vi "log.write.vi"(4 "Channel":string, 6 "Arguments":map{string, string}(c390), 7 "Time Stamp (now: system time)":timestamp format="%<%x %.3X>T", 8 "error in":errorcluster, 9 "Message":string, 10 "dataSourceRid":string, 11 "Nominal Client in":refnum<class "Nominal Client.lvclass">) -> (0 "error out":errorcluster, 3 "Nominal Client out":refnum<class "Nominal Client.lvclass">)   [LabVIEW 2020, in "Nominal Client.lvclass"]
doc: "Synchronously writes logs to a Nominal data source.\n\nMessage (required, string) The log content describing the event. Can include placeholder tokens for dynamic values.\n\nArguments (optional)\nKey-value pairs providing structured context data or filling message placeholders.\n\nChannel (optional, string, defaults to \"logs\") Logical grouping to organize logs by source, type, or system component for filtering and analysis."
uses:
  Nominal Client.lvclass
  <vilib>/Utility/error.llb/Error Cluster From Error Code.vi
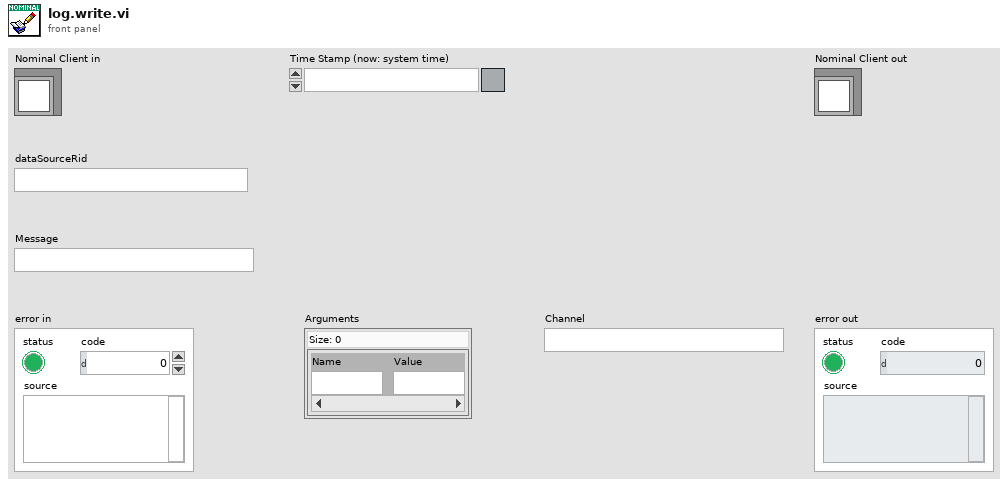
[diagram p1: front panel]
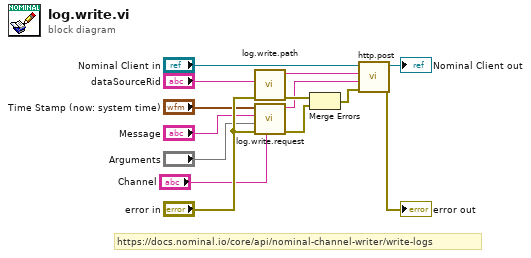
[diagram p0: block diagram]
diagram:
  # "https://docs.nominal.io/core/api/nominal-channel-writer/write-logs"
  n1 = call "log.write.path.vi"("error in"="error in", "dataSourceRid"="dataSourceRid") -> ("error out"=w5:errorcluster, "path"=w11:string)  [unwired: 8 in]
  n2 = call "log.write.request.vi"("Channel"="Channel", "error in"="error in", "Arguments"="Arguments", "Message"="Message", "Time Stamp (now: system time)"="Time Stamp (now: system time)") -> ("error out"=w4:errorcluster, "request"=w2:string)  [unwired: 5 in]
  n3 = Merge Errors(w5, w4) -> (w3:errorcluster)
  n4 = call "http.post.vi"("error in"=w3, "Request body"=w2, "Path"=w11, "Nominal Client in"="Nominal Client in") -> ("error out"=→"error out":errorcluster, "Nominal Client out"=→"Nominal Client out":refnum<class "Nominal Client.lvclass">)  [unwired: 4 in, 2 out]
